vi "AssignDirections.vi"(8 "Actual Angle":dbl, 11 "Target Angle":dbl) -> (0 "Reverse Wheel Direction":bool, 2 "Lowest Angle Error":dbl, 3 "Turn Clockwise":bool)   [LabVIEW 2013, in "ProcessorHelperFunctions.lvlib"]
uses:
  ProcessorHelperFunctions.lvlib
panel:
  out "Error CCW Rev":dbl
  out "Error CW Rev":dbl
  out "Error CCW No Rev":dbl
  out "Error CW No Rev":dbl
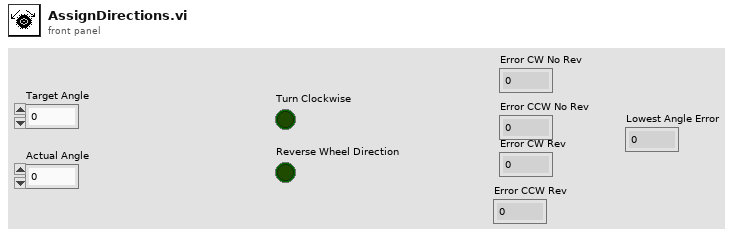
[diagram p1: front panel]
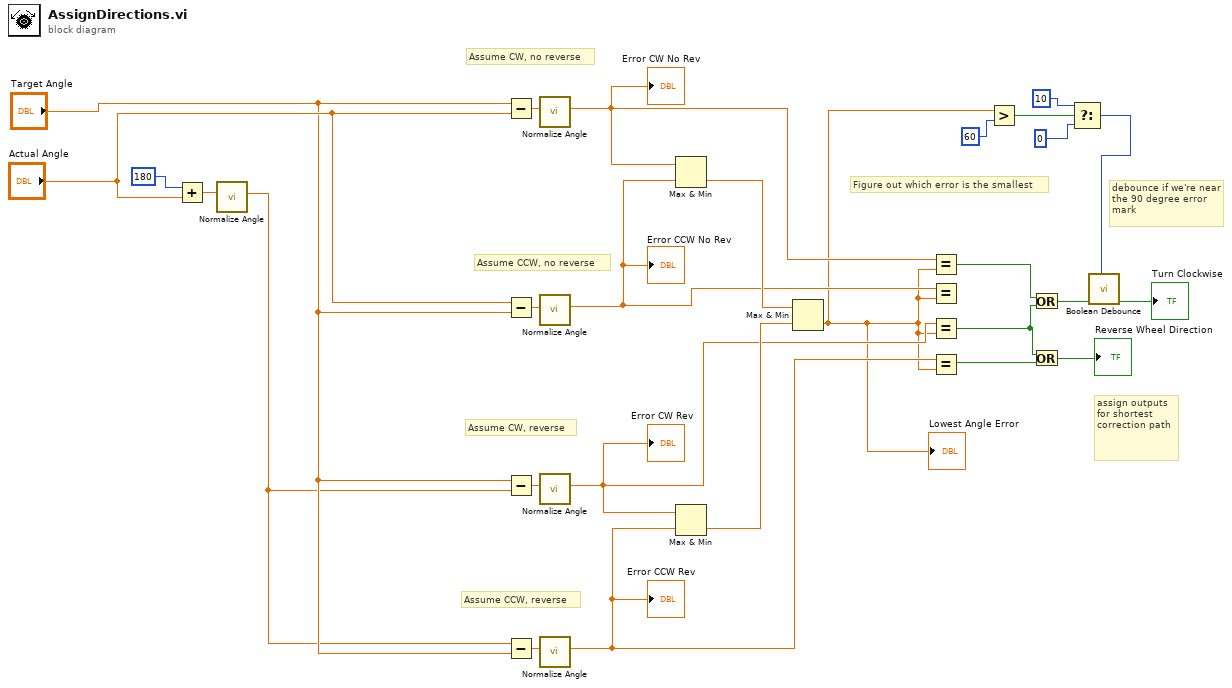
[diagram p0: block diagram]
diagram:
  # "debounce if we're near the 90 degree error mark"
  # "assign outputs for shortest correction path"
  # "Figure out which error is the smallest"
  # "Assume CCW, reverse"
  # "Assume CW, reverse"
  # "Assume CCW, no reverse"
  # "Assume CW, no reverse"
  n1 = Add(x=180, y="Actual Angle") -> (x+y=w23:dbl)
  n2 = call "Normalize Angle.vi"("Input"=w23) -> ("Output"=w19:dbl)  [unwired: 10 in]
  n3 = Subtract(x="Target Angle", y="Actual Angle") -> (x-y=w27:dbl)
  n4 = Subtract(x="Actual Angle", y="Target Angle") -> (x-y=w26:dbl)
  n5 = Subtract(x="Target Angle", y=w19) -> (x-y=w22:dbl)
  n6 = Subtract(x=w19, y="Target Angle") -> (x-y=w21:dbl)
  n7 = call "Normalize Angle.vi"("Input"=w27) -> ("Output"=w16:dbl)  [unwired: 10 in]
  "Error CW No Rev" <- w16
  n8 = call "Normalize Angle.vi"("Input"=w26) -> ("Output"=w15:dbl)  [unwired: 10 in]
  "Error CCW No Rev" <- w15
  n9 = call "Normalize Angle.vi"("Input"=w22) -> ("Output"=w14:dbl)  [unwired: 10 in]
  "Error CW Rev" <- w14
  n10 = call "Normalize Angle.vi"("Input"=w21) -> ("Output"=w13:dbl)  [unwired: 10 in]
  "Error CCW Rev" <- w13
  n11 = Max & Min(x=w16, y=w15) -> (min(x,y)=w18:dbl)  [unwired: 1 out]
  n12 = Max & Min(x=w14, y=w13) -> (min(x,y)=w17:dbl)  [unwired: 1 out]
  n13 = Max & Min(x=w18, y=w17) -> (min(x,y)=w5:dbl)  [unwired: 1 out]
  "Lowest Angle Error" <- w5
  n14 = Equal?(x=w16, y=w5) -> (x = y?=w12:bool)
  n15 = Equal?(x=w15, y=w5) -> ()  [unwired: 1 out]
  n16 = Equal?(x=w14, y=w5) -> (x = y?=w10:bool)
  n17 = Equal?(x=w13, y=w5) -> (x = y?=w9:bool)
  n18 = Greater?(x=w5, y=60) -> (0:w2:bool)
  n19 = Or(x=w12, y=w10) -> (x .or. y?=w7:bool)
  n20 = Or(x=w10, y=w9) -> (x .or. y?=→"Reverse Wheel Direction":bool)
  n21 = Select(t=10, s=w2, f=0) -> (s? t:f=w1:i32)
  n22 = call "Boolean Debounce.vi"("loops"=w1, "input"=w7) -> ("output"=→"Turn Clockwise":bool)  [unwired: 9 in]
